vi "Step 4 - Model and Simulate FXP Decimation (MRate).vi"() -> ()   [LabVIEW 2023]
doc: "Demonstrates how to use the DFD FXP MRate Modeling VI to model a fixed-point decimation filter, the DFD FXP MRate Simulation VI to simulate the filtering process, and the DFD MRate Filtering VI to get the reference floating-point filtering results.\n\nThis example uses the DFD FXP MRate Modeling VI to create a model of the fixed-point decimation filter. The example then uses the DFD FXP MRate Simulation VI to apply the fixed-point decimation filter model to a signal from the Uniform White Noise VI and simulates the filtering result. To verify the simulation, this example also uses the DFD MRate Filtering VI to filter the same signal that the Uniform White Noise VI generates with the original reference floating-point decimation filter and finally uses the MSE VI to compute the mean squared error (MSE) of the two filtered signals.\n\nAfter you run the VI, compare the signal from the reference floating-point decimation filter and the signal from the fixed-point decimation filter model. The ideal result is that the two signals overlap each other."
uses:
  <vilib>/addons/Digital Filter Design/_Objects.llb/DFD Coef Norm Type.ctl
  <vilib>/addons/Digital Filter Design/FXPMRateSim.llb/DFD FXP MRate Simulation (DBL).vi
  <vilib>/addons/Digital Filter Design/Multirate.llb/DFD MRate Filtering (Array).vi
  <vilib>/addons/Digital Filter Design/NI_DigFilterLicensed.lvlib
  <vilib>/Analysis/NI_AALPro.lvlib
  <vilib>/Analysis/NI_AALBase.lvlib
panel:
  out "MSE":dbl format="%.3g"
  out "Filtered Signals":dbl[][](graph)
  # "Select Help>>Show Context Help and move the cursor over the VI icon for more information."
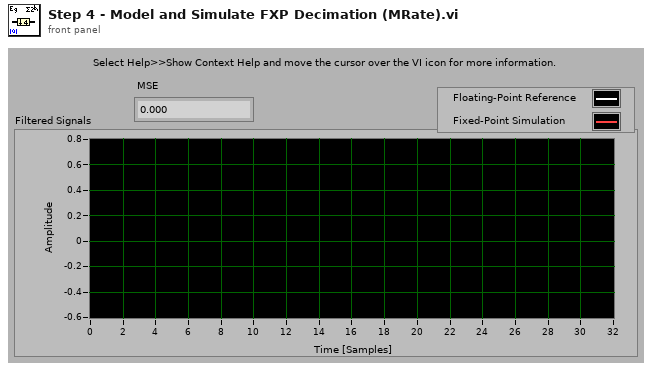
[diagram p1: front panel]
types:
  T1 = typedef "NI_DigFilterLicensed.lvlib/DFD Coef Norm Type.ctl" = enum16{"No Norm", "Time Domain 1-Norm", "Time Domain 2-Norm", "Time Domain Inf-Norm"}
  T2 = typedef "NI_DigFilterLicensed.lvlib/DFD Multirate Filter Obj.ctl" = cluster{"mMRate_Structure":enum16{"CIC", "FIR", "IIR", "Lattice"}, "mMRate_Mode":T3, "mMRate_Factor":i32, "mMRate_FIRParams":cluster{"mMRate_FIR_H":dbl[], "mMRate_FIR_IsNyquist?":bool, "mMRate_FIR_IsSymmetric?":bool}, "mMRate_CICParams":cluster{"mMRate_CIC_#Stage":i32, "mMRate_CIC_Lag":i32, "mMRate_CIC_Type":enum16{"Lowpass", "Highpass"}}, "mMRate_Order":i32, "mMRate_Version":string, "mMRate_Comments":string, "mMRate_RationalFactor":cluster{"mMRate_L":i32, "mMRate_M":i32}, "mMRate_Fs":dbl, "mMRate_Quantized?":bool, "mMRate_QFilterGain":dbl, "mMRate_CoefWl":i16, "mMRate_Scaling":cluster{"mMRate_ScaleByPowerOf2?":bool, "mMRate_ScaleType":T1}, "mMRate_InputWl":i16, "mMRate_OutputWl":i16, "mMRate_OutputMode":T4, "mMRate_MultMode":T5, "mMRate_BitPruning":bool, "mMRate_GainWl":i16, "mMRate_OutputFwl":i16, "mMRate_SumIwl":i16, "mMRate_InputIwl ":i16, "mMRate_SumWl":i16, "mMRate_CoefIwl":i16}
  T3 = typedef "NI_DigFilterLicensed.lvlib/DFD Multirate Mode.ctl" = i16
  T4 = typedef "NI_DigFilterLicensed.lvlib/DFD Round-off Mode.ctl" = enum16{"Nearest", "Truncation"}
  T5 = typedef "NI_DigFilterLicensed.lvlib/DFD FXP MRate Multiply Mode.ctl" = enum16{"Truncated", "Full"}
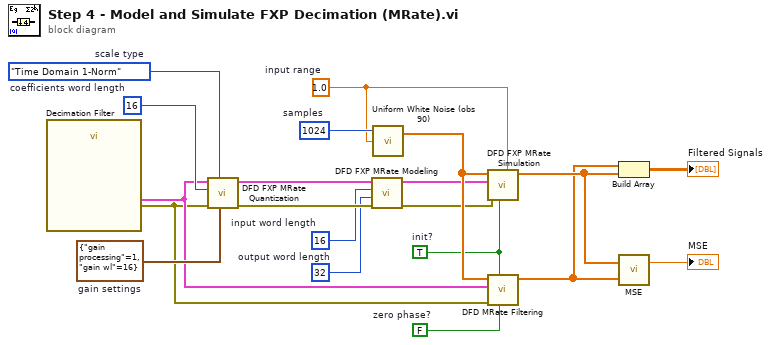
[diagram p0: block diagram]
diagram:
  w3 = i16 32  # output word length
  w4 = i16 16  # input word length
  w18 = i16 16  # coefficients word length
  w6 = cluster{"gain processing":u16, "gain wl":i16} {"gain processing"=1, "gain wl"=16}  # gain settings
  w9 = 1.0  # input range
  w13 = FALSE  # zero phase?
  w5 = TRUE  # init?
  w17 = 1024  # samples
  w20 = DFD_Coef_Norm_Type."Time Domain 1-Norm"  # scale type
  n1 = call "Decimation Filter"() -> ("error out"=w1:errorcluster, "multirate filter out"=w2:T2)  [unwired: 10 out]
  n2 = call <vilib>:"DFD FXP MRate Quantization.vi"("gain settings"=w6, "scale type"=w20, "error in (no error)"=w1, "coefficients word length"=w18, "multirate filter in"=w2) -> ("error out"=w8:errorcluster, "multirate filter out"=w19:T2)  [unwired: 1 in, 4 out]
  n3 = call <vilib>:"DFD FXP MRate Modeling.vi"("error in (no error)"=w8, "output word length"=w3, "input word length"=w4, "multirate filter in"=w19) -> ("error out"=w7:errorcluster, "multirate filter out"=w15:T2)  [unwired: 4 in, 2 out]
  n4 = call <vilib>:"Uniform White Noise (obs 90).vi"("amplitude"=w9, "samples"=w17) -> ("uniform white noise"=w16:dbl[])  [unwired: 1 in, 1 out]
  n5 = call-poly <vilib>:"DFD FXP MRate Simulation.vi"("input range"=w9, "init? (T)"=w5, "error in (no error)"=w7, "multirate filter"=w15, "signal in"=w16) -> ("DBL signal out"=w12:dbl[])  [unwired: 6 out]
  n6 = call-poly <vilib>:"DFD MRate Filtering.vi"("zero phase? (T)"=w13, "init? (F)"=w5, "error in (no error)"=w1, "multirate filter"=w2, "signal in"=w16) -> ("signal out"=w11:dbl[])  [unwired: 6 out]
  n7 = Build Array(w11, w12) -> (→"Filtered Signals":dbl[][])
  n8 = call <vilib>:"MSE.vi"("X Values"=w11, "Y Values"=w12) -> ("mse"=→"MSE":dbl)  [unwired: 1 out]
